vi "Conditional Tunnels.vi"() -> ()   [LabVIEW 2015]
panel:
  out "Random Numbers < 0.5":dbl[](array[numeric])
  out "Random Numbers > 0.5":dbl[](array[numeric])
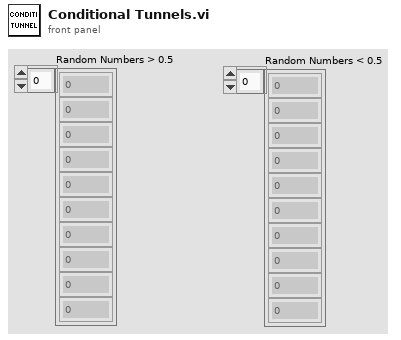
[diagram p1: front panel]
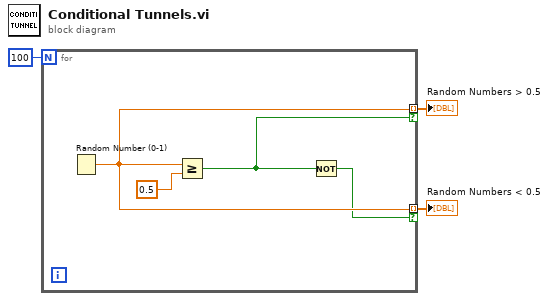
[diagram p0: block diagram]
diagram:
  n1 = for {
    N: 100 -> [_]
    tunnel: [w6] -> w3 mode=indexing if=w5
    tunnel: [w6] -> w2 mode=indexing if=w4
    n2 = Random Number (0-1)() -> (number: 0 to 1=w6:dbl)
    n3 = Greater Or Equal?(x=w6, y=0.5) -> (x >= y?=w5:bool)
    n4 = Not(x=w5) -> (.not. x?=w4:bool)
  }
  "Random Numbers > 0.5" <- w3
  "Random Numbers < 0.5" <- w2
